vi "ATTN.vi"(8 "error in (no error)":errorcluster, 10 "Attn":u32(ring) items=["Off", "On"], 11 "VISA resource name":refnum<visa-resource-name>) -> (0 "error out":errorcluster, 3 "VISA resource name out":refnum<visa-resource-name>)   [LabVIEW 2013, in "Newport 1830-C.lvlib"]
doc: "Attenuator\n0=OFF\n1=ON"
uses:
  Newport 1830-C.lvlib
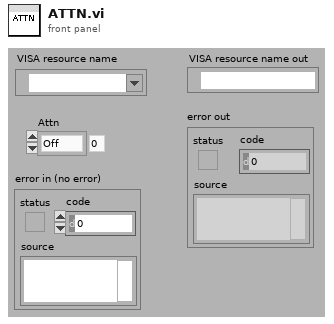
[diagram p1: front panel]
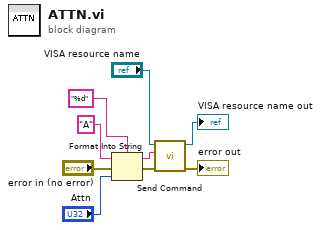
[diagram p0: block diagram]
diagram:
  n1 = Format Into String(format string="%d", initial string="A" ("command"), error in="error in (no error)", "Attn") -> (resulting string=w3:string, error out=w5:errorcluster)
  n2 = call "Send Command.vi"("error in (no error)"=w5, "write buffer"=w3, "VISA resource name In"="VISA resource name") -> ("error out"=→"error out":errorcluster, "VISA resource name out"=→"VISA resource name out":refnum<visa-resource-name>)  [unwired: 7 in]
